vi "Read Status Notifier.vi"(8 "error in (no error)":errorcluster, 11 "Message in":refnum<class "Message.lvclass">) -> (0 "error out":errorcluster, 1 "nb en attente":i32, 2 "latest notification":variant, 3 "Message out":refnum<class "Message.lvclass">)   [LabVIEW 2015, in "Message.lvclass"]
uses:
  Message.lvclass
  Message.lvclass/Message.ctl
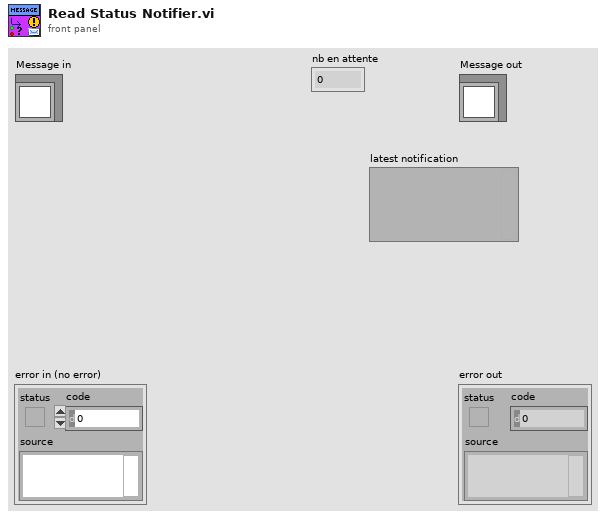
[diagram p1: front panel]
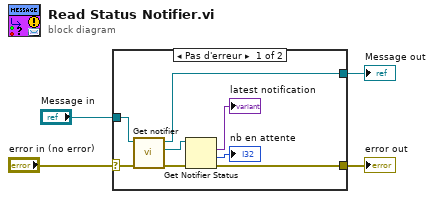
[diagram p0: block diagram]
diagram:
  n1 = case shown="Pas d'erreur" "error in (no error)" {
    selector: "error in (no error)" -> [w11 w14]
    tunnel: [w8 w14] -> w3
    tunnel: [w10 w13] -> w1
    tunnel: "Message in" -> [w12 w13]
    frame No Error {
      n2 = call "Get notifier.vi"("error in (no error)"=w11, "Message en entrée"=w12) -> ("error out"=w9:errorcluster, "notifier"=w7:refnum<notifier>, "Message en sortie"=w10:refnum<class "Message.lvclass">)  [unwired: 7 in]
      n3 = Get Notifier Status(notifier=w7, error in (no error)=w9) -> (current notification=→"latest notification":variant, # waiting=→"nb en attente":i32, error out=w8:errorcluster)  [unwired: 2 out]
    }
    frame Error {
    }
  }
  "error out" <- w3
  "Message out" <- w1
